vi "LookupTableSelection.vi"(8 "Error In":errorcluster, 11 "LookupTableParam":refnum<vi>) -> (0 "Error Out":errorcluster)   [LabVIEW 2015]
uses:
  Controls/LookupTableParam.ctl
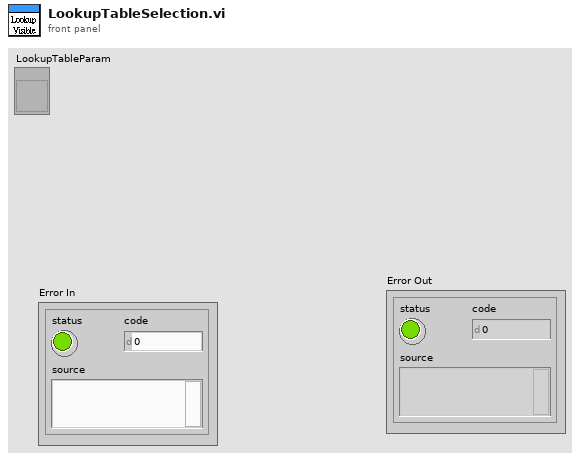
[diagram p1: front panel]
types:
  T1 = typedef "LookupTableParam.ctl" = cluster{"Function":enum16{"Equalizer", "Reverse", "Logarithmic", "Exponential", "Square", "Square Root", "Power X", "Power 1/X"}, "Power Value":sgl}
  T2 = enum16{"Equalizer", "Reverse", "Logarithmic", "Exponential", "Square", "Square Root", "Power X", "Power 1/X"}
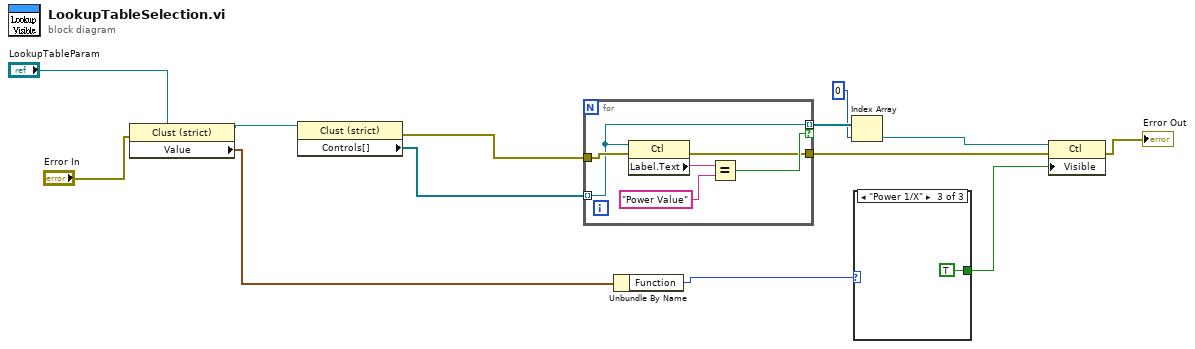
[diagram p0: block diagram]
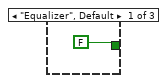
[diagram p2: hidden frame]
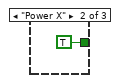
[diagram p3: hidden frame]
diagram:
  n1 = property class="Clust (strict)"(reference="LookupTableParam", error in="Error In") -> (reference out=w10:refnum<vi>, "Value"=w8:T1)  [unwired: 1 out]
  n2 = property class="Clust (strict)"(reference=w10) -> (error out=w12:errorcluster, "Controls[]"=w13:refnum<vi>[])  [unwired: 1 in, 1 out]
  n3 = for {
    tunnel: w13 -> [w16] mode=indexing
    tunnel: w12 -> [w17]
    tunnel: [w16] -> w7 mode=indexing if=w15
    tunnel: [w14] -> w2
    n4 = property class="Ctl"(reference=w16, error in=w17) -> (error out=w14:errorcluster, "Label.Text"=w19:string)  [unwired: 1 out]
    n5 = Equal?(x=w19, y="Power Value") -> (x = y?=w15:bool)
  }
  n6 = Unbundle By Name(w8) -> ("Function"=w4:T2)
  n7 = Index Array(array=w7, index=0) -> (element=w5:refnum<vi>)
  n8 = case shown="\"Power 1/X\"" w4 {
    tunnel: [FALSE ("Visible") TRUE ("Visible") TRUE ("Visible")] -> w3
    frame "Equalizer", Default {
    }
    frame "Power X" {
    }
    frame "Power 1/X" {
    }
  }
  n9 = property class="Ctl"(reference=w5, error in=w2, "Visible"=w3) -> (error out=→"Error Out":errorcluster)  [unwired: 1 out]
